vi "SaveDictionnaire.vi"(8 "error in (no error)":errorcluster, 11 "Dictionnaire":T1) -> (0 "error out":errorcluster)   [LabVIEW 2013]
uses:
  Dictionnaire.ctl
  CleValeur.ctl
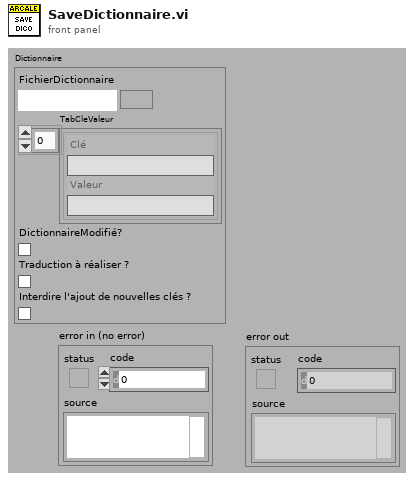
[diagram p1: front panel]
types:
  T1 = typedef "Dictionnaire.ctl" = cluster{"FichierDictionnaire":path, "TabCleValeur":T2[], "DictionnaireModifié?":bool, "Traduction à réaliser ?":bool, "Interdire l'ajout de nouvelles clés ?":bool}
  T2 = typedef "CleValeur.ctl" = cluster{"Clé":string, "Valeur":string}
  T3 = enum16{"open", "replace", "create", "open or create", "replace or create", "replace or create with confirmation"}
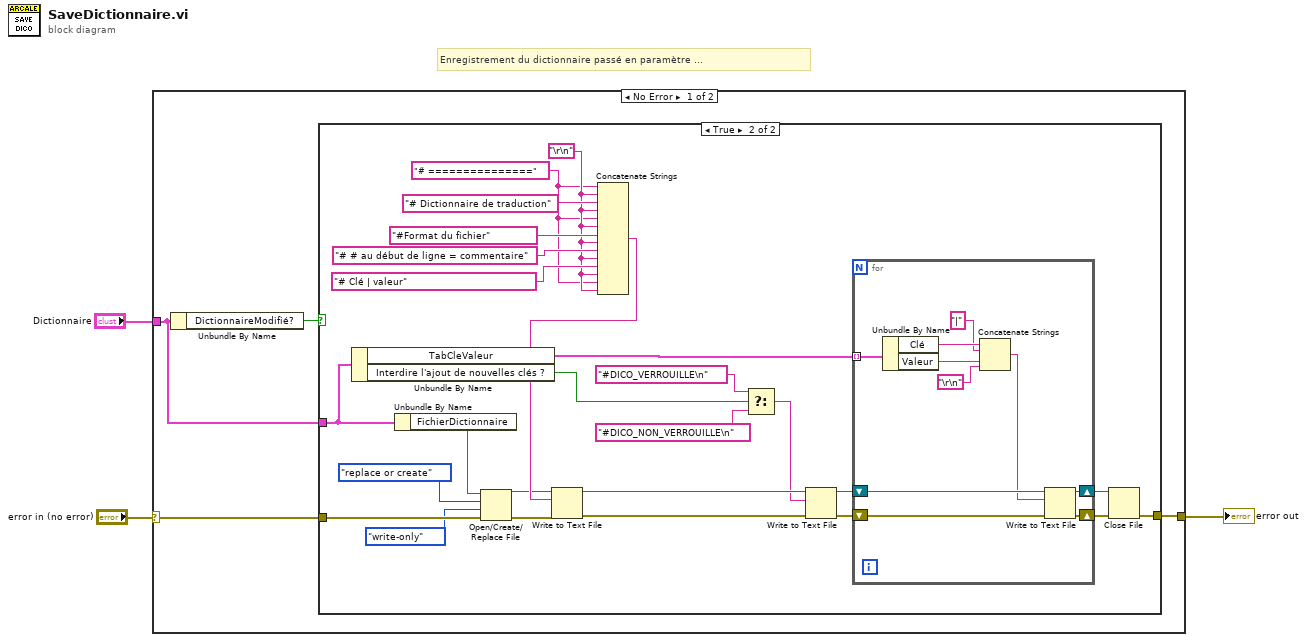
[diagram p0: block diagram]
diagram:
  # "Enregistrement du dictionnaire passé en paramètre ..."
  n1 = case shown="No Error" "error in (no error)" {
    selector: "error in (no error)" -> [w7 w45]
    tunnel: [w6 w45] -> w2
    tunnel: "Dictionnaire" -> [w5 _]
    frame No Error {
      n2 = Unbundle By Name(w5) -> ("DictionnaireModifié?"=w4:bool)
      n3 = case shown="True" w4 {
        tunnel: w7 -> [w8 w34]
        tunnel: [w8 w18] -> w6
        tunnel: w5 -> [_ w17]
        frame False {
          # "Il n'y a rien à modifier ...."
        }
        frame True {
          w25 = "\r\n"
          w24 = "# ===============" ("string")
          n4 = Unbundle By Name(w17) -> ("TabCleValeur"=w21:T2[], "Interdire l'ajout de nouvelles clés ?"=w12:bool)
          n5 = Unbundle By Name(w17) -> ("FichierDictionnaire"=w33:path)
          n6 = Open/Create/Replace File(file path (use dialog)=w33, error in=w34, operation (0:open)=T3."replace or create", access (0:read/write)=enum16{"read/write", "read-only", "write-only"}."write-only") -> (refnum out=w22:refnum<file>, error out=w30:errorcluster)  [unwired: 2 in, 1 out]
          n7 = Concatenate Strings(w24, w25, "# Dictionnaire de traduction" ("string"), w25, w24, w25, "#Format du fichier" ("string"), w25, "# # au début de ligne = commentaire" ("string"), w25, "# Clé | valeur" ("string"), w25, w24, w25) -> (w23:string)
          n8 = Write to Text File(file (use dialog)=w22, text=w23, error in=w30) -> (refnum out=w16:refnum<file>, error out=w14:errorcluster)  [unwired: 1 in, 1 out]
          n9 = Select(t="#DICO_VERROUILLE\n", s=w12, f="#DICO_NON_VERROUILLE\n") -> (s? t:f=w11:string)
          n10 = Write to Text File(file (use dialog)=w16, text=w11, error in=w14) -> (refnum out=w15:refnum<file>, error out=w13:errorcluster)  [unwired: 1 in, 1 out]
          n11 = for {
            tunnel: w21 -> [w44] mode=indexing
            shift-right: [w38] -> w19
            shift-left: w13 -> [w39]
            shift-right: [w37] -> w20
            shift-left: w15 -> [w36]
            n12 = Unbundle By Name(w44) -> ("Clé"=w43:string, "Valeur"=w42:string)
            n13 = Concatenate Strings(w43, "|", w42, "\r\n") -> (w35:string)
            n14 = Write to Text File(file (use dialog)=w36, text=w35, error in=w39) -> (refnum out=w37:refnum<file>, error out=w38:errorcluster)  [unwired: 1 in, 1 out]
          }
          n15 = Close File(refnum=w20, error in=w19) -> (error out=w18:errorcluster)  [unwired: 1 out]
        }
      }
    }
    frame Error {
    }
  }
  "error out" <- w2
